vi "Read N Images from Buffer.vi"(8 "error in":errorcluster, 9 "timeout (-1 = wait forever)":i32 format="%d ms", 10 "count (-1 = all)":i32=-1, 11 "IMAQdx Triggered Continuous Acquisition in":refnum<class "IMAQdx Triggered Continuous Acquisition.lvclass">) -> (0 "error out":errorcluster, 2 "Images":refnum<class "Generic Image.lvclass">[](array[class]), 3 "IMAQdx Triggered Continuous Acquisition out":refnum<class "IMAQdx Triggered Continuous Acquisition.lvclass">)   [LabVIEW 2024, in "IMAQdx Triggered Continuous Acquisition.lvclass"]
uses:
  IMAQdx Triggered Continuous Acquisition.lvclass
  Source/Typedefs/Generic Image/Generic Image.lvclass
  IMAQdx Triggered Continuous Acquisition.lvclass/IMAQdx Triggered Continuous Acquisition.ctl
  Base/IMAQdx Base Configure Strategy.lvclass
  <vilib>/vision/driver/NI_Vision_Acquisition_Software.lvlib
  <vilib>/vision/driver/IMAQdx.llb/IMAQdx Buffer Number Mode.ctl
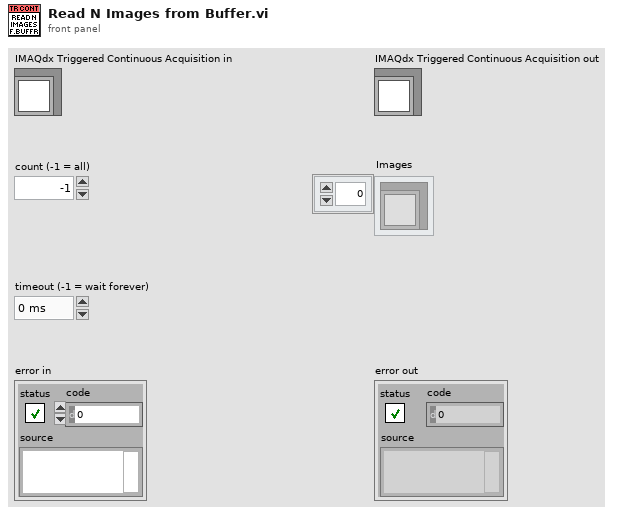
[diagram p1: front panel]
types:
  T1 = typedef "Generic Image.lvclass/Pixel Format.ctl" = enum16{"Grayscale (U8)", "Grayscale (I16)", "Grayscale (SGL)", "Complex (CSG)", "RGB (U32)", "HSL (U32)", "RGB (U64)", "Grayscale (U16)"}
  T2 = typedef "IMAQdx.ctl" = refnum<k21>
  T3 = typedef "NI_Vision_Acquisition_Software.lvlib/IMAQdx Buffer Number Mode.ctl" = enum32{"Next", "Last", "Buffer Number", "Every", "Last New"}
  T4 = typedef "IMAQ Image.ctl" = refnum<image>
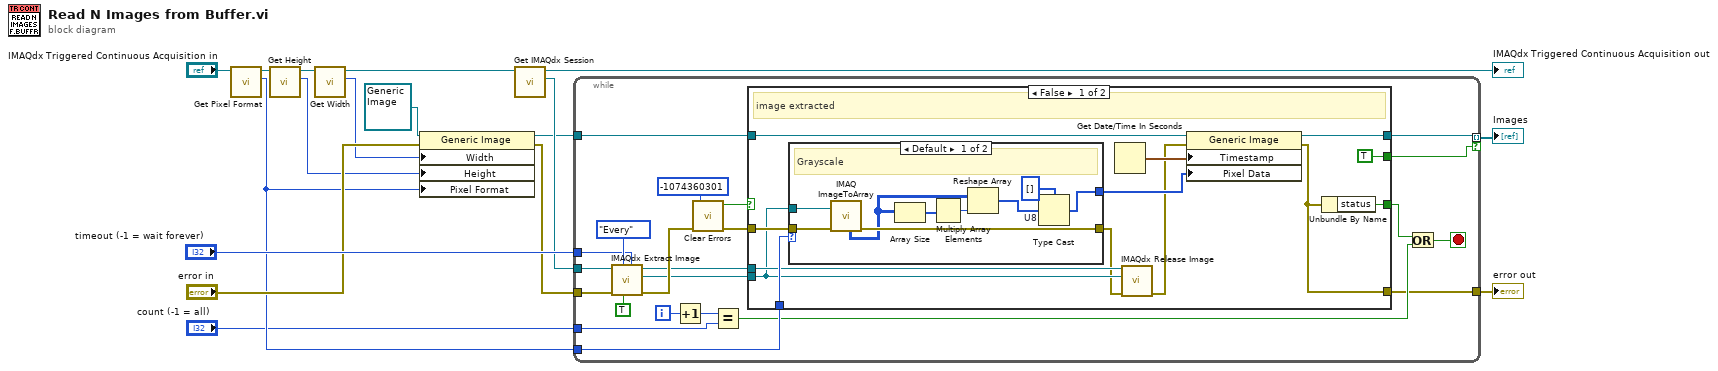
[diagram p0: block diagram]
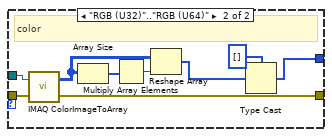
[diagram p2: hidden frame]
diagram:
  n1 = call "Get Pixel Format.vi"("IMAQdx Base Configure Strategy in"="IMAQdx Triggered Continuous Acquisition in") -> ("Pixel Format"=w2:T1, "IMAQdx Base Configure Strategy out"=w11:refnum<class "IMAQdx Triggered Continuous Acquisition.lvclass">)  [unwired: 9 in]
  n2 = call "Get Height.vi"("IMAQdx Base Configure Strategy in"=w11) -> ("Height"=w4:i32, "IMAQdx Base Configure Strategy out"=w10:refnum<class "IMAQdx Triggered Continuous Acquisition.lvclass">)  [unwired: 9 in]
  n3 = call "Get Width.vi"("IMAQdx Base Configure Strategy in"=w10) -> ("Width"=w5:i32, "IMAQdx Base Configure Strategy out"=w9:refnum<class "IMAQdx Triggered Continuous Acquisition.lvclass">)  [unwired: 9 in]
  n4 = property class="Generic Image"(reference=refnum<class "Generic Image.lvclass"> refnum ("Generic Image.lvclass"), error in="error in", "Width"=w5, "Height"=w4, "Pixel Format"=w2) -> (reference out=w3:refnum<class "Generic Image.lvclass">, error out=w6:errorcluster)
  n5 = call "Get IMAQdx Session.vi"("IMAQdx Base Configure Strategy in"=w9) -> ("IMAQdx Session"=w12:T2, "IMAQdx Base Configure Strategy out"=→"IMAQdx Triggered Continuous Acquisition out":refnum<class "IMAQdx Triggered Continuous Acquisition.lvclass">)  [unwired: 9 in]
  n6 = while {
    tunnel: w12 -> [w39]
    tunnel: w6 -> [w38]
    tunnel: [w19] -> w14
    tunnel: [w33] -> w15 mode=indexing if=w26
    tunnel: w3 -> [w34]
    tunnel: "timeout (-1 = wait forever)" -> [w32]
    tunnel: w2 -> [w30]
    tunnel: "count (-1 = all)" -> [w20]
    i -> [w23]
    stop <- w24 stop-if-true
    n7 = call <vilib>:"IMAQdx Extract Image.vi"("Timeout (ms)"=w32, "Release Previous (true)"=TRUE, "Buffer Number Mode (Next)"=IMAQdx_Buffer_Number_Mode."Every", "error in"=w38, "Session In"=w39) -> ("error out"=w35:errorcluster, "Image Out"=w31:T4, "Session Out"=w25:T2)  [unwired: 3 in, 1 out]
    n8 = Increment(x=w23) -> (x+1=w21:i32)
    n9 = call <vilib>:"Clear Errors.vi"("error in (no error)"=w35, "specific error code to clear (0: all)"=-1074360301) -> ("error out"=w29:errorcluster, "specific error cleared?"=w27:bool)  [unwired: 4 in]
    n10 = Equal?(x=w21, y=w20) -> (x = y?=w22:bool)
    n11 = case shown="False" w27 {
      selector: w27 -> [_ w71]
      tunnel: w34 -> [w52 w72]
      tunnel: [w51 w72] -> w33
      tunnel: w31 -> [w44 _]
      tunnel: w30 -> [w49 _]
      tunnel: [w41 w73] -> w19
      tunnel: w29 -> [w47 w73]
      tunnel: [TRUE _] -> w26
      tunnel: w25 -> [w45 _]
      tunnel: [w40 w71] -> w18
      frame False {
        # "image extracted"
        n12 = case shown="Default" w49 {
          tunnel: w47 -> [w61 w69]
          tunnel: [w60 w68] -> w43
          tunnel: w44 -> [w59 w70]
          tunnel: [w55 w62] -> w48
          frame Default {
            w56 = u8[] []  # U8
            # "Grayscale"
            n13 = call "IMAQ ImageToArray"("error in (no error)"=w61, "Image"=w59) -> ("Image Pixels (U16)"=w53:u16[][], "error out"=w60:errorcluster)  [unwired: 2 in, 3 out]
            n14 = Array Size(array=w53) -> (size(s)=w57:i32[])
            n15 = Multiply Array Elements(1:w57) -> (0:w58:i32)
            n16 = Reshape Array(w53, w58) -> (w54:u16[])
            n17 = Type Cast(type=w56, x=w54) -> (*(type *) &x=w55:u8[])
          }
          frame "RGB (U32)".."RGB (U64)" {
            # "color"
            n18 = call "IMAQ ColorImageToArray"("Image"=w70, "error in (no error)"=w69) -> ("Image Pixels (U32)"=w65:u32[][], "error out"=w68:errorcluster)  [unwired: 2 in, 1 out]
            n19 = Array Size(array=w65) -> (size(s)=w66:i32[])
            n20 = Multiply Array Elements(1:w66) -> (0:w67:i32)
            n21 = Reshape Array(w65, w67) -> (w64:u32[])
            n22 = Type Cast(type=u8[] [], x=w64) -> (*(type *) &x=w62:u8[])
          }
        }
        n23 = Get Date/Time In Seconds() -> (seconds since 1Jan1904=w50:timestamp)
        n24 = call <vilib>:"IMAQdx Release Image.vi"("error in"=w43, "Image"=w44, "Session In"=w45) -> ("error out"=w42:errorcluster)  [unwired: 7 in, 1 out]
        n25 = property class="Generic Image"(reference=w52, error in=w42, "Timestamp"=w50, "Pixel Data"=w48) -> (reference out=w51:refnum<class "Generic Image.lvclass">, error out=w41:errorcluster)
        n26 = Unbundle By Name(w41) -> ("status"=w40:bool)
      }
      frame True {
        # "no image extracted"
      }
    }
    n27 = Or(x=w18, y=w22) -> (x .or. y?=w24:bool)
  }
  "error out" <- w14
  "Images" <- w15
